vi "Manual Adjust Voltage.vi"(8 "error in (no error)":errorcluster, 10 "VISA resource name":refnum<visa-resource-name>, 11 "Supply Voltage:":string(combo)) -> (0 "error out":errorcluster, 2 "L2 Adjusted":string, 3 "L1 Adjusted":string)   [LabVIEW 2020]
uses:
  Trunk/Utility/Custom Pallet Controls/Custom Pallet DBL.ctl
  Trunk/Utility/Custom Pallet Controls/Custom Pallet Forward.ctl
  Type Definition/Chroma Driver Select.ctl
panel:
  out "Description":string="Manually Adjust Voltage\n(If Needed)"
  in  "Tab Control":enum32{"Page 1", "Page 2"}(tab)
  out "Adjusted Output":string[](array[string])
  in  "Complete":T1
  in  "Chroma L2 (Volts)":T2 format="%.1f"
  in  "Chroma L1 (Volts)":T2 format="%.1f"
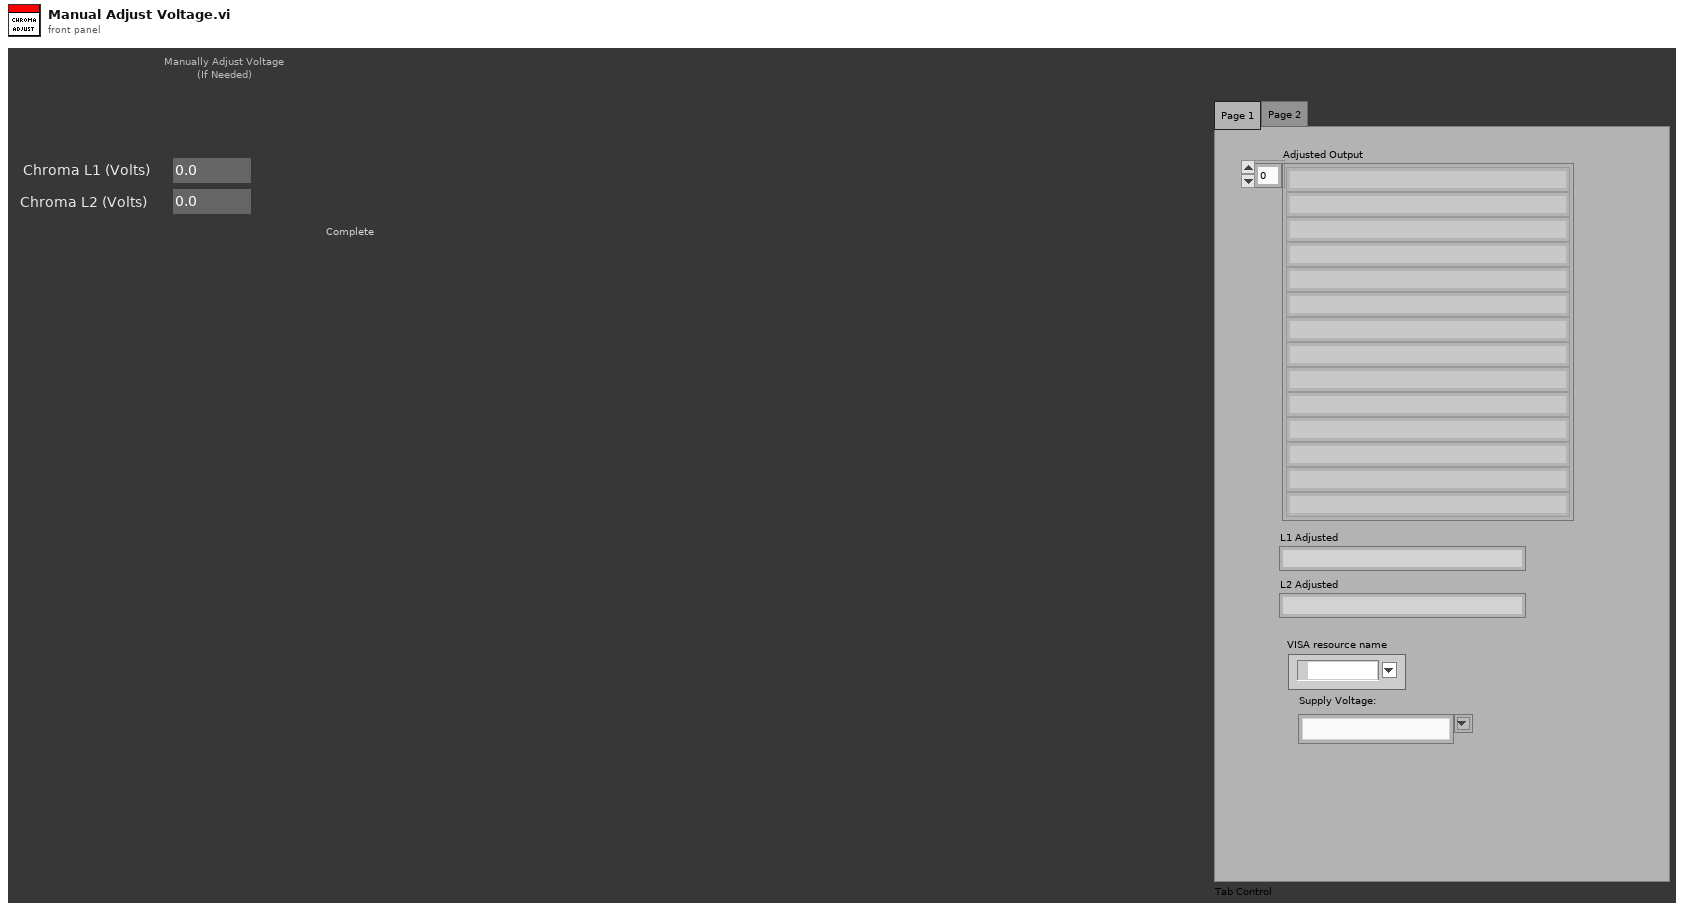
[diagram p1: front panel]
types:
  T1 = typedef "Custom Pallet Forward.ctl" = bool
  T2 = typedef "Custom Pallet DBL.ctl" = dbl
  T3 = typedef "Chroma Driver Select.ctl" = enum16{"Initialize", "Output On 120", "Output On 240", "Output On 208", "Output Off", "Status", "Send Command", "Track Current"}
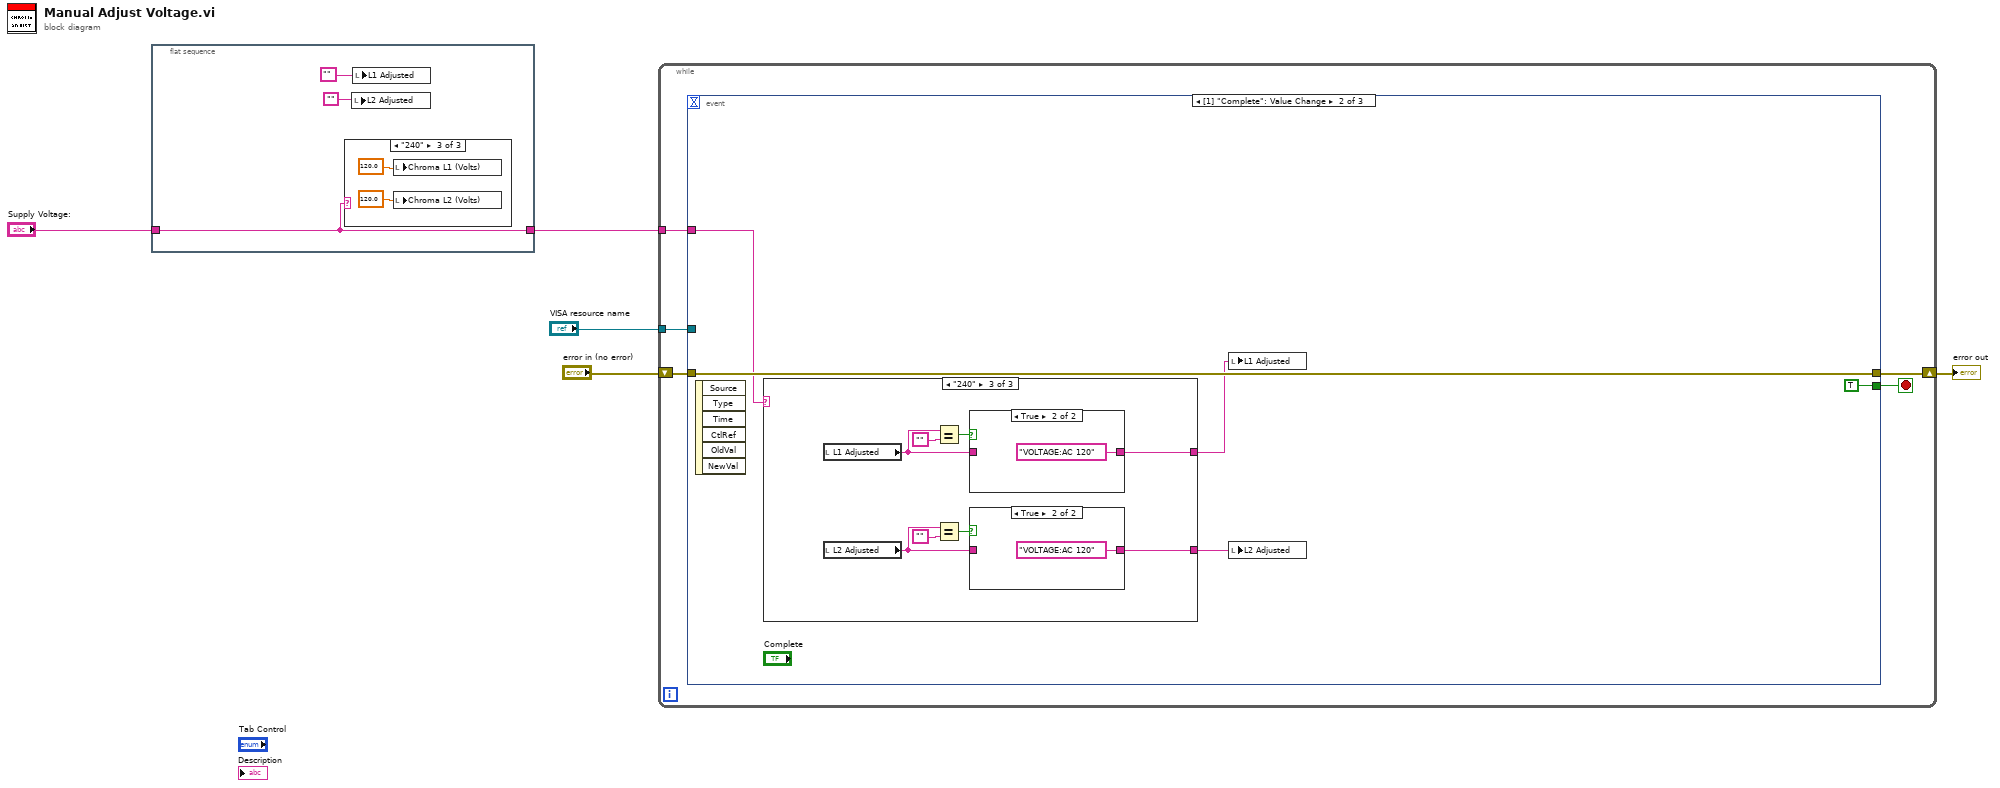
[diagram p0: block diagram]
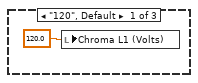
[diagram p2: hidden frame]
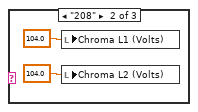
[diagram p3: hidden frame]
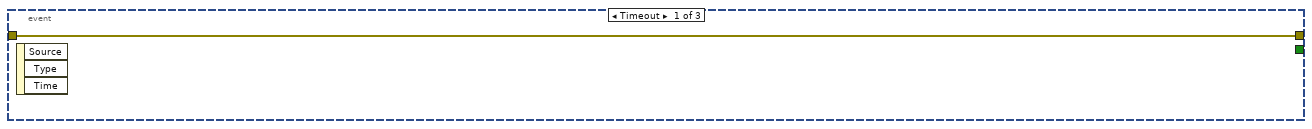
[diagram p4: hidden frame]
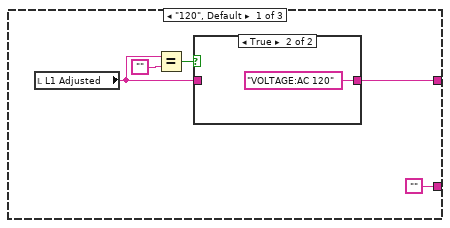
[diagram p5: hidden frame]
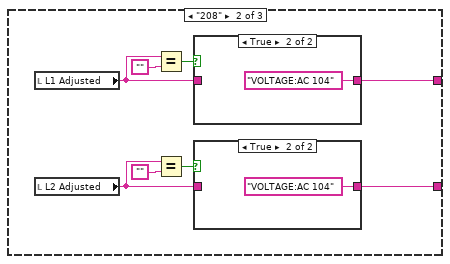
[diagram p7: hidden frame]
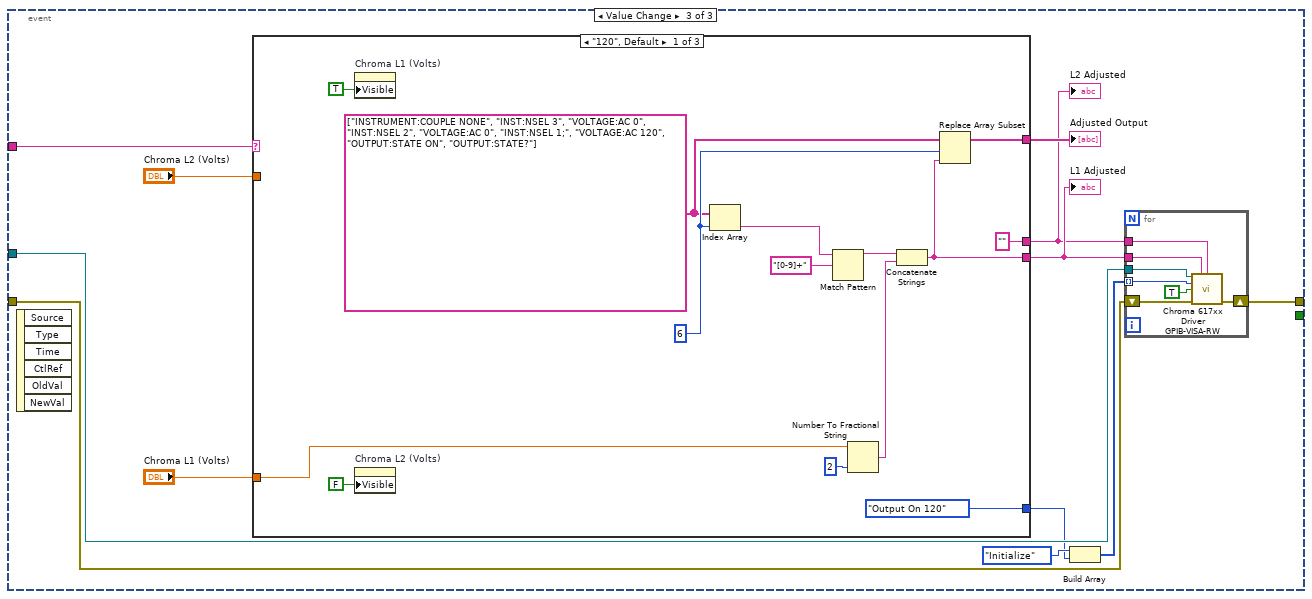
[diagram p12: hidden frame]
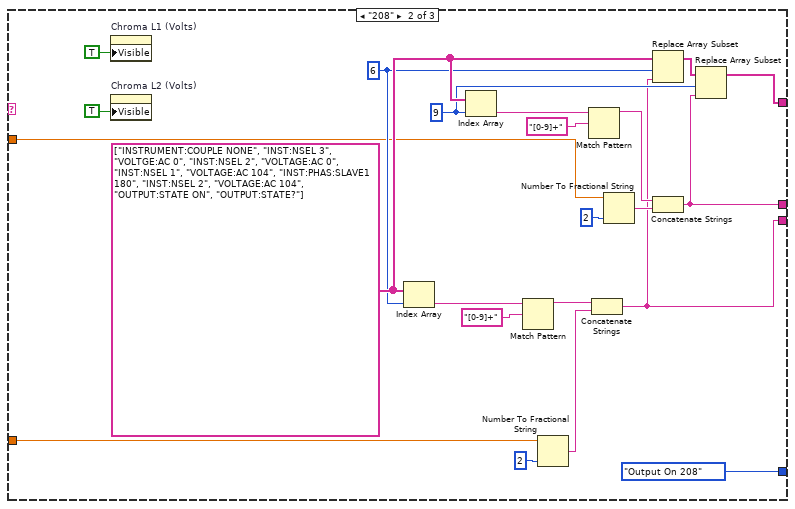
[diagram p13: hidden frame]
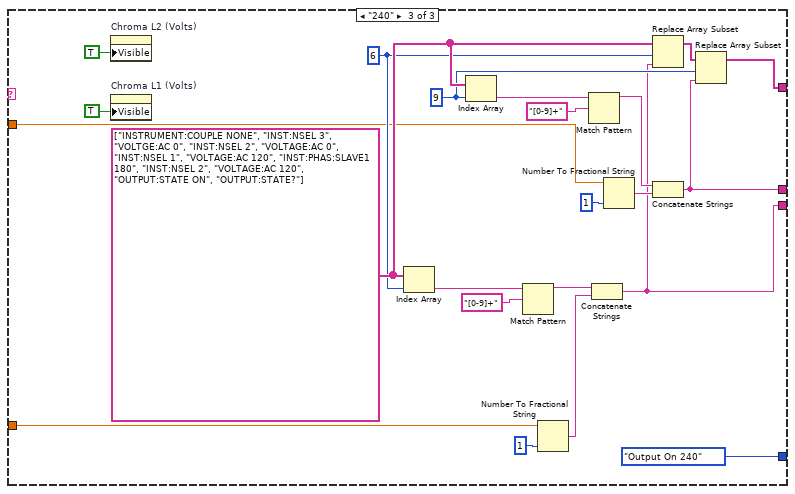
[diagram p14: hidden frame]
diagram:
  n1 = flat-sequence {
    tunnel: "Supply Voltage:" -> [w8]
    tunnel: [w8] -> w1
    frame #0 {
      n2 = case shown="\"240\"" w8 {
        frame "120", Default {
          n3 = local write "Chroma L1 (Volts)"(T2 120.0 ("Chroma L1 (Volts)")) -> ()
        }
        frame "208" {
          n4 = local write "Chroma L1 (Volts)"(T2 104.0 ("Chroma L1 (Volts)")) -> ()
          n5 = local write "Chroma L2 (Volts)"(T2 104.0 ("Chroma L2 (Volts)")) -> ()
        }
        frame "240" {
          n6 = local write "Chroma L1 (Volts)"(T2 120.0 ("Chroma L1 (Volts)")) -> ()
          n7 = local write "Chroma L2 (Volts)"(T2 120.0 ("Chroma L2 (Volts)")) -> ()
        }
      }
      n8 = local write "L2 Adjusted"("") -> ()
      n9 = local write "L1 Adjusted"("") -> ()
    }
  }
  n10 = while {
    tunnel: w1 -> [w18]
    tunnel: "VISA resource name" -> [w17]
    shift-right: [w15] -> w3
    shift-left: "error in (no error)" -> [w16]
    stop <- w14 stop-if-true
    n11 = event shown="[1] \"Complete\": Value Change" {
      selector: _ -> [_ _ _]
      dyn-events: _ -> [_ _ _]
      timeout: _ -> [_ _ _]
      tunnel: w18 -> [_ w22 w67]
      tunnel: w17 -> [_ _ w66]
      tunnel: w16 -> [w19 w23 w65]
      tunnel: [w19 w23 w64] -> w15
      tunnel: [_ TRUE _] -> w14
      event Timeout {
        n12 = event-data() -> ()  [unwired: 1 in, 3 out]
      }
      event Value Change {
        n13 = event-data() -> ()  [unwired: 1 in, 6 out]
        n14 = case shown="\"240\"" w22 {
          tunnel: [w26 w35 w45] -> w21
          tunnel: ["" w33 w44] -> w20
          frame "120", Default {
            n15 = local read "L1 Adjusted"() -> (w27:string)
            n16 = Equal?(x=w27, y="") -> (x = y?=w29:bool)
            n17 = case shown="True" w29 {
              tunnel: [w30 "VOLTAGE:AC 120"] -> w26
              tunnel: w27 -> [w30 _]
              frame False {
              }
              frame True {
              }
            }
          }
          frame "208" {
            n18 = local read "L1 Adjusted"() -> (w34:string)
            n19 = local read "L2 Adjusted"() -> (w32:string)
            n20 = Equal?(x=w34, y="") -> (x = y?=w37:bool)
            n21 = Equal?(x=w32, y="") -> (x = y?=w38:bool)
            n22 = case shown="True" w37 {
              tunnel: [w40 "VOLTAGE:AC 104"] -> w35
              tunnel: w34 -> [w40 _]
              frame False {
              }
              frame True {
              }
            }
            n23 = case shown="True" w38 {
              tunnel: [w42 "VOLTAGE:AC 104"] -> w33
              tunnel: w32 -> [w42 _]
              frame False {
              }
              frame True {
              }
            }
          }
          frame "240" {
            n24 = local read "L1 Adjusted"() -> (w47:string)
            n25 = local read "L2 Adjusted"() -> (w46:string)
            n26 = Equal?(x=w47, y="") -> (x = y?=w49:bool)
            n27 = Equal?(x=w46, y="") -> (x = y?=w50:bool)
            n28 = case shown="True" w49 {
              tunnel: [w52 "VOLTAGE:AC 120"] -> w45
              tunnel: w47 -> [w52 _]
              frame False {
              }
              frame True {
              }
            }
            n29 = case shown="True" w50 {
              tunnel: [w54 "VOLTAGE:AC 120"] -> w44
              tunnel: w46 -> [w54 _]
              frame False {
              }
              frame True {
              }
            }
          }
        }
        n30 = local write "L1 Adjusted"(w21) -> ()
        n31 = local write "L2 Adjusted"(w20) -> ()
      }
      event Value Change {
        n32 = event-data() -> ()  [unwired: 1 in, 6 out]
        n33 = case shown="\"120\", Default" w67 {
          tunnel: "Chroma L2 (Volts)" -> [_ w96 w118]
          tunnel: "Chroma L1 (Volts)" -> [w82 w95 w117]
          tunnel: [w81 w94 w116] -> w63
          tunnel: [w77 w91 w113] -> w62
          tunnel: ["" w90 w112] -> w61
          tunnel: [Chroma_Driver_Select."Output On 120" ("Chroma Power Select") Chroma_Driver_Select."Output On 208" ("Chroma Power Select") Chroma_Driver_Select."Output On 240" ("Chroma Power Select")] -> w57
          frame "120", Default {
            w80 = string[] ["INSTRUMENT:COUPLE NONE", "INST:NSEL 3", "VOLTAGE:AC 0", "INST:NSEL 2", "VOLTAGE:AC 0", "INST:NSEL 1;", "VOLTAGE:AC 120", "OUTPUT:STATE ON", "OUTPUT:STATE?"]
            w88 = 6 ("index")
            n34 = property on="Chroma L1 (Volts)" class="DigNum (strict)"("Visible"=TRUE) -> ()  [unwired: 2 in, 2 out]
            n35 = property on="Chroma L2 (Volts)" class="DigNum (strict)"("Visible"=FALSE) -> ()  [unwired: 2 in, 2 out]
            n36 = Index Array(array=w80, index=w88) -> (element=w84:string)
            n37 = Match Pattern(string=w84, regular expression="[0-9]+") -> (before substring=w85:string)  [unwired: 1 in, 3 out]
            n38 = Number To Fractional String(number=w82, precision (6)=i16 2) -> (F-format string=w86:string)  [unwired: 2 in]
            n39 = Concatenate Strings(w85, w86) -> (w77:string)
            n40 = Replace Array Subset(array=w80, new element=w77, index=w88) -> (w81:string[])
          }
          frame "208" {
            w108 = 9 ("index")
            w107 = 6 ("index")
            w109 = string[] ["INSTRUMENT:COUPLE NONE", "INST:NSEL 3", "VOLTGE:AC 0", "INST:NSEL 2", "VOLTAGE:AC 0", "INST:NSEL 1", "VOLTAGE:AC 104", "INST:PHAS:SLAVE1 180", "INST:NSEL 2", "VOLTAGE:AC 104", "OUTPUT:STATE ON", "OUTPUT:STATE?"]
            n41 = property on="Chroma L1 (Volts)" class="DigNum (strict)"("Visible"=TRUE) -> ()  [unwired: 2 in, 2 out]
            n42 = property on="Chroma L2 (Volts)" class="DigNum (strict)"("Visible"=TRUE) -> ()  [unwired: 2 in, 2 out]
            n43 = Index Array(array=w109, index=w107) -> (element=w98:string)
            n44 = Index Array(array=w109, index=w108) -> (element=w100:string)
            n45 = Match Pattern(string=w98, regular expression="[0-9]+") -> (before substring=w101:string)  [unwired: 1 in, 3 out]
            n46 = Number To Fractional String(number=w95, precision (6)=i16 2) -> (F-format string=w102:string)  [unwired: 2 in]
            n47 = Match Pattern(string=w100, regular expression="[0-9]+") -> (before substring=w106:string)  [unwired: 1 in, 3 out]
            n48 = Concatenate Strings(w101, w102) -> (w91:string)
            n49 = Number To Fractional String(number=w96, precision (6)=i16 2) -> (F-format string=w105:string)  [unwired: 2 in]
            n50 = Replace Array Subset(array=w109, new element=w91, index=w107) -> (w110:string[])
            n51 = Concatenate Strings(w106, w105) -> (w90:string)
            n52 = Replace Array Subset(array=w110, new element=w90, index=w108) -> (w94:string[])
          }
          frame "240" {
            w130 = 9 ("index")
            w129 = 6 ("index")
            w131 = string[] ["INSTRUMENT:COUPLE NONE", "INST:NSEL 3", "VOLTGE:AC 0", "INST:NSEL 2", "VOLTAGE:AC 0", "INST:NSEL 1", "VOLTAGE:AC 120", "INST:PHAS:SLAVE1 180", "INST:NSEL 2", "VOLTAGE:AC 120", "OUTPUT:STATE ON", "OUTPUT:STATE?"]
            n53 = property on="Chroma L2 (Volts)" class="DigNum (strict)"("Visible"=TRUE) -> ()  [unwired: 2 in, 2 out]
            n54 = property on="Chroma L1 (Volts)" class="DigNum (strict)"("Visible"=TRUE) -> ()  [unwired: 2 in, 2 out]
            n55 = Index Array(array=w131, index=w129) -> (element=w120:string)
            n56 = Index Array(array=w131, index=w130) -> (element=w122:string)
            n57 = Match Pattern(string=w120, regular expression="[0-9]+") -> (before substring=w123:string)  [unwired: 1 in, 3 out]
            n58 = Number To Fractional String(number=w117, precision (6)=i16 1) -> (F-format string=w124:string)  [unwired: 2 in]
            n59 = Match Pattern(string=w122, regular expression="[0-9]+") -> (before substring=w128:string)  [unwired: 1 in, 3 out]
            n60 = Concatenate Strings(w123, w124) -> (w113:string)
            n61 = Number To Fractional String(number=w118, precision (6)=i16 1) -> (F-format string=w127:string)  [unwired: 2 in]
            n62 = Replace Array Subset(array=w131, new element=w113, index=w129) -> (w132:string[])
            n63 = Concatenate Strings(w128, w127) -> (w112:string)
            n64 = Replace Array Subset(array=w132, new element=w112, index=w130) -> (w116:string[])
          }
        }
        "L1 Adjusted" <- w62
        "Adjusted Output" <- w63
        "L2 Adjusted" <- w61
        n65 = Build Array(Chroma_Driver_Select."Initialize" ("Chroma Power Select"), w57) -> (w56:T3[])
        n66 = for {
          tunnel: w66 -> [w74]
          tunnel: w62 -> [w70]
          tunnel: w61 -> [w69]
          shift-right: [w72] -> w64
          shift-left: w65 -> [w73]
          tunnel: w56 -> [w68] mode=indexing
          n67 = call "Chroma 617xx Driver GPIB-VISA-RW.vi"("VISA resource name"=w74, "L1 Adjusted"=w70, "L2 Adjusted"=w69, "Chroma Power Select"=w68, "Use Adjusted Voltage"=TRUE, "error in (no error)"=w73) -> ("error out"=w72:errorcluster)  [unwired: 8 in, 1 out]
        }
      }
    }
  }
  "error out" <- w3
